vi "CAN Jaguar Close.vi"(8 "error in (no error)":errorcluster, 11 "CAN Jaguar Ref":T1={"Device Number"=0, "Control Mode"=enum."Percent VBus", "Inverted"=FALSE, "Semaphore"=refnum, "Max Vout"=12.0, "DevStatus"={"status"=FALSE, "code"=0, "source"=""}}) -> (0 "error out":errorcluster)   [LabVIEW 2009, in "CAN.lvlib"]
uses:
  CAN.lvlib
  SubVIs/CAN Jaguar Ref.ctl
  SubVIs/CAN Jaguar Control Mode.ctl
  SubVIs/CAN Motor Message IDs.ctl
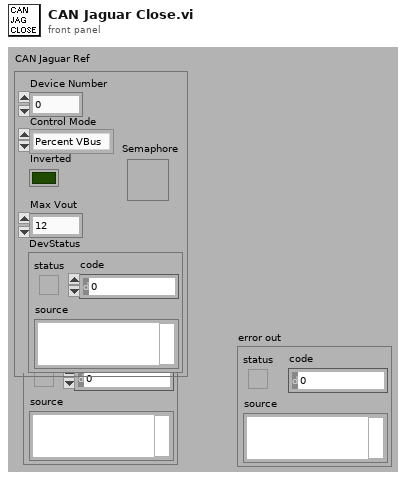
[diagram p1: front panel]
types:
  T1 = typedef "CAN.lvlib/CAN Jaguar Ref.ctl" = cluster{"Device Number":u8, "Control Mode":T2, "Inverted":bool, "Semaphore":T3, "Max Vout":dbl, "DevStatus":errorcluster}
  T2 = typedef "CAN.lvlib/CAN Jaguar Control Mode.ctl" = enum16{"Percent VBus", "Speed", "Position", "Current"}
  T3 = typedef "Semaphore RefNum" = refnum<k1>
  T4 = typedef "CAN.lvlib/CAN Motor Message IDs.ctl" = u32
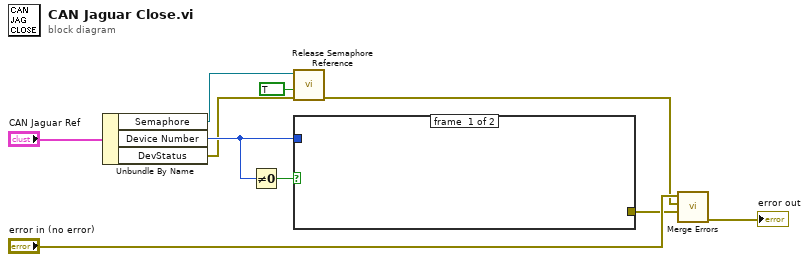
[diagram p0: block diagram]
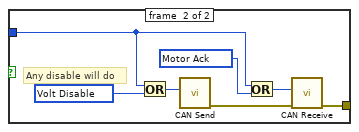
[diagram p2: hidden frame]
diagram:
  n1 = Unbundle By Name("CAN Jaguar Ref") -> ("Semaphore"=w1:T3, "Device Number"=w5:u8, "DevStatus"=w3:errorcluster)
  n2 = Not Equal To 0?(x=w5) -> (x != 0?=w6:bool)
  n3 = call <vilib>:"Release Semaphore Reference.vi"("error in (no error)"=w3, "force destroy? (F)"=TRUE, "semaphore"=w1) -> ("error out"=w2:errorcluster)  [unwired: 8 out]
  n4 = case shown="True" w6 {
    tunnel: w5 -> [_ w12]
    tunnel: [_ w11] -> w7
    frame #0 {
    }
    frame #1 {
      w17 = T4 33693696 items=["Volt Enable"=33685504, "Volt Disable"=33685568, "Volt Set"=33685632, "Volt Set Ramp"=33685696, "Speed Enable"=33686528, "Speed Disable"=33686592, "Speed Set"=33686656, "Speed P"=33686720, "Speed I"=33686784, "Speed D"=33686848, "Speed Ref"=33686912, "Position Enable"=33688576, "Position Disable"=33688640, "Position Set"=33688704, "Position P"=33688768, "Position I"=33688832, "Position D"=33688896, "Position Ref"=33688960, "Current Enable"=33689600, "Current Disable"=33689664, "Current Set"=33689728, "Current P"=33689792, "Current I"=33689856, "Current D"=33689920, "Status VOut"=33690624, "Status VBus"=33690688, "Status Current"=33690752, "Status Temp"=33690816, "Status Position"=33690880, "Status Speed"=33690944, "Status Limit"=33691008, "Status Fault"=33691072, "Status Power"=33691136, "Config Num Brushes"=33692672, "Config Encoder Lines"=33692736, "Config Pot Turns"=33692800, "Config Brake Coast"=33692864, "Config Limit Mode"=33692928, "Config Limit Fwd"=33692992, "Config Limit Rev"=33693056, "Config Max VOut"=33693120, "Config Fault Time"=33693184, "Motor Ack"=33693696] ("CAN Motor Message IDs")
      w14 = T4 33685568 items=["Volt Enable"=33685504, "Volt Disable"=33685568, "Volt Set"=33685632, "Volt Set Ramp"=33685696, "Speed Enable"=33686528, "Speed Disable"=33686592, "Speed Set"=33686656, "Speed P"=33686720, "Speed I"=33686784, "Speed D"=33686848, "Speed Ref"=33686912, "Position Enable"=33688576, "Position Disable"=33688640, "Position Set"=33688704, "Position P"=33688768, "Position I"=33688832, "Position D"=33688896, "Position Ref"=33688960, "Current Enable"=33689600, "Current Disable"=33689664, "Current Set"=33689728, "Current P"=33689792, "Current I"=33689856, "Current D"=33689920, "Status VOut"=33690624, "Status VBus"=33690688, "Status Current"=33690752, "Status Temp"=33690816, "Status Position"=33690880, "Status Speed"=33690944, "Status Limit"=33691008, "Status Fault"=33691072, "Status Power"=33691136, "Config Num Brushes"=33692672, "Config Encoder Lines"=33692736, "Config Pot Turns"=33692800, "Config Brake Coast"=33692864, "Config Limit Mode"=33692928, "Config Limit Fwd"=33692992, "Config Limit Rev"=33693056, "Config Max VOut"=33693120, "Config Fault Time"=33693184, "Motor Ack"=33693696] ("CAN Motor Message IDs")
      # "Any disable will do"
      n5 = Or(x=w12, y=w14) -> (x .or. y?=w15:T4)
      n6 = call "CAN Send.vi"("messageID"=w15) -> ("error out"=w13:errorcluster)  [unwired: 2 in, 8 out]
      n7 = Or(x=w12, y=w17) -> (x .or. y?=w16:T4)
      n8 = call "CAN Receive.vi"("error in (no error)"=w13, "Message ID"=w16) -> ("error out"=w11:errorcluster)  [unwired: 1 in, 8 out]
    }
  }
  n9 = call <vilib>:"Merge Errors.vi"("error in 3 (no error)"=w7, "error in 2 (no error)"=w2, "error in 1 (no error)"="error in (no error)") -> ("error out"=→"error out":errorcluster)  [unwired: 1 in, 3 out]
